vi "signed value to slide format (subVI).vi"(8 "error in (no error)":errorcluster, 10 "value":dbl, 11 "slide refnum":refnum<vi>) -> (0 "error out":errorcluster, 3 "slide refnum out":refnum<vi>)   [LabVIEW 2021]
panel:
  in  "zero range (+/-0.1)":dbl=0.1
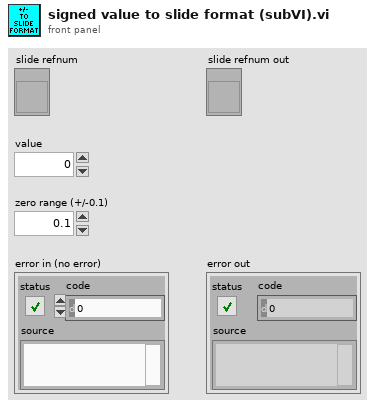
[diagram p1: front panel]
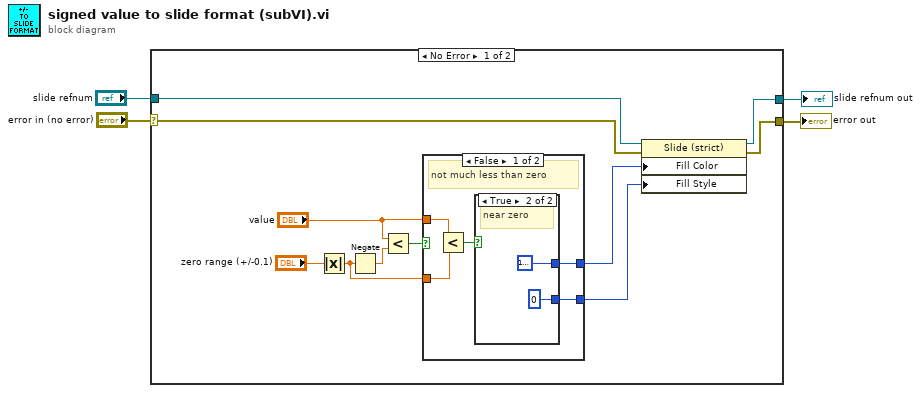
[diagram p0: block diagram]
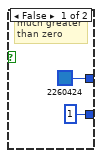
[diagram p2: hidden frame]
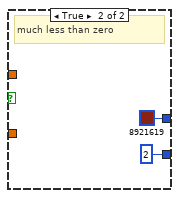
[diagram p3: hidden frame]
diagram:
  n1 = case shown="No Error" "error in (no error)" {
    selector: "error in (no error)" -> [w13 w28]
    tunnel: [w14 w28] -> w4
    tunnel: [w12 w27] -> w2
    tunnel: "slide refnum" -> [w11 w27]
    frame No Error {
      n2 = Absolute Value(x="zero range (+/-0.1)") -> (abs(x)=w7:dbl)
      n3 = Negate(x=w7) -> (-x=w8:dbl)
      n4 = Less?(x="value", y=w8) -> (x < y?=w15:bool)
      n5 = case shown="False" w15 {
        tunnel: [w20 2 ("Fill Style")] -> w9
        tunnel: w7 -> [w19 _]
        tunnel: "value" -> [w18 _]
        tunnel: [w16 u32 8921619 ("Fill Color")] -> w5
        frame False {
          # "not much less than zero"
          n6 = Less?(x=w18, y=w19) -> (x < y?=w17:bool)
          n7 = case shown="True" w17 {
            tunnel: [1 ("Fill Style") 0 ("Fill Style")] -> w20
            tunnel: [u32 2260424 ("Fill Color") u32 16777216 ("Fill Color")] -> w16
            frame False {
              # "much greater than zero"
            }
            frame True {
              # "near zero"
            }
          }
        }
        frame True {
          # "much less than zero"
        }
      }
      n8 = property on="Property Node" class="Slide (strict)"(reference=w11, error in=w13, "Fill Color"=w5, "Fill Style"=w9) -> (reference out=w12:refnum<vi>, error out=w14:errorcluster)
    }
    frame Error {
    }
  }
  "slide refnum out" <- w2
  "error out" <- w4
